vi "basic - Loopback.vi"() -> ()   [LabVIEW 2020]
uses:
  src/AIM664LV.lvlib
  src/_polimorphicInstances/session/Fdx Close Session (Port).vi
  src/_polimorphicInstances/control/Fdx Start (Rx).vi
  src/_polimorphicInstances/session/Fdx Create Session (RX-Monitor).vi
  src/_polimorphicInstances/session/Fdx Create Session (Tx-Generic).vi
  src/_polimorphicInstances/control/Fdx Start (Tx).vi
  src/_polimorphicInstances/control/Fdx Stop (Tx).vi
  src/_polimorphicInstances/control/Fdx Stop (Rx).vi
  src/_controls/session_monitor_config.ctl
  src/_controls/queue_header_generic.ctl
panel:
  out "current time":timestamp
  out "tx timed out":bool
  out "rx timed out":bool
  in  "Data":u8[](array[numeric])=[3, 0, 0, 0, 0, 0, 2, 0, 0, 1, 1, 32, 8, 0, 69, 0, 0, 45, 0, 0, 64, 0, 1, 17, 141, 223, 10, 1, 1, 0, 224, 224, 0, 0, 0, 1, 0, 2, 0, 25, 0, 0, 65, 66, 67, 68, 69, 70, 71, 72, 73, 74, 75, 76, 77, 78, 79, 80, 81, 11] format="%x"
  in  "HeaderInfo":T1={"InterFrameGap"=1000, "PacketGroupWaitTime"=10000, "PayloadBufferMode"=0, "PayloadGenerationMode"=0, "PreambleCount"=0, "Skew"=1, "NetSelect"=4, "FrameStartMode"=1, "PhysErrorInjection"=0, "SequenceNumberInit"=65535, "SequenceNumberOffset"=65535} {"NetSelect" items=["FDX_TX_FRAME_DLY_A"=0, "FDX_TX_FRAME_DLY_B"=1, "FDX_TX_FRAME_BOTH "=3, "FDX_TX_FRAME_ONLY_A"=4, "FDX_TX_FRAME_ONLY_B "=5]; "FrameStartMode" items=["FDX_TX_FRAME_START_IFG", "FDX_TX_FRAME_START_PGWT", "FDX_TX_FRAME_START_TRG"]; "PhysErrorInjection" items=["FDX_TX_FRAME_ERR_OFF"=0, "FDX_TX_FRAME_ERR_CRC"=1, "FDX_TX_FRAME_ERR_ALI"=2, "FDX_TX_FRAME_ERR_PRE"=4, "FDX_TX_FRAME_ERR_PHY"=8]; "SequenceNumberInit" items=["FDX_TX_FRAME_SEQ_INIT_AUTO"=65535]; "SequenceNumberOffset" items=["FDX_TX_FRAME_SEQ_OFFS_AUTO "=65535]; "PayloadGenerationMode" items=["FDX_TX_FRAME_PGM_USER"=0, "FDX_TX_FRAME_PGM_IP_PART"=1, "FDX_TX_FRAME_PGM_IP_FULL"=2, "FDX_TX_FRAME_PGM_IP_PART_TT"=10, "FDX_TX_FRAME_PGM_IP_FULL_TT"=20]; "PayloadBufferMode" items=["FDX_TX_FRAME_PBM_STD", "FDX_TX_FRAME_PBM_MAC", "FDX_TX_FRAME_PBM_UDP"]}
  out "error out":errorcluster
  out "QueueReadOut":T2 {"ReadBuffer" format="%.0x"}
  in  "EntryCount (1)":u32=5
  out "MonStatus":T3 {"MonStatus" items=["FDX_MON_OFF", "FDX_MON_WAIT_FOR_TRIGGER", "FDX_MON_TRIGGERED", "FDX_MON_STOPPED", "FDX_MON_FULL", "FDX_MON_OVERLOAD"]}
  out "GlobalStat Out":T4
  in  "Control":u32(ring)=1 items=["FDX_RX_GS_RES_NO_CNT", "FDX_RX_GS_RES_ALL_CNT", "FDX_RX_GS_RES_ERR_CNT"]
  out "TxStatus":T5
  out "rx link ok":bool
  out "tx link ok":bool
  out "GlobMonSize":u32
  in  "RecordingFileName":path
  in  "MaxFileSize MB (1)":u32=1
  in  "Strobe":u32(ring) items=["FDX_MON_STROBE_DIS", "FDX_MON_STROBE_STOP", "FDX_MON_STROBE_START"]
  in  "CaptureMode":u32(ring) items=["FDX_MON_SINGLE ", "FDX_MON_CONTINUOUS", "FDX_MON_SELECTIVE", "FDX_MON_RECORDING", "FDX_MON_REROS", "FDX_MON_HMU"]
  in  "TriggerPosition":u32
  in  "MonitorConfig":T6 {"DefaultCronoMode" items=["FDX_RX_DEFAULT_ENA_CNT", "FDX_RX_DEFAULT_MON_ENA_ALL", "FDX_RX_DEFAULT_MON_ENA_GOOD"]}
  in  "Rx Port":u32=1
  in  "Rx Board":u32
  out "PortInitOut":T7 {"PortConfig" items=["FDX_SINGLE", "FDX_REDUNDANT"]}
  out "TxQueueInfo":cluster{"QueueBaseAddr":u32, "QueueSizeOut":u32}
  in  "Tx Board":u32
  in  "QueueSizeIn":u32
  in  "Tx Port":u32
  # "ARINC 664 Loopback"
  # "Overview: This examples helps to setup the board (or boards) and validate that it can send and receive parameters.\n\nRequirement: One AIM ARINC-664 board with installed AIM ARINC 664 BSP.\nRestrictions: None.\nInstruction:\n1. Select the Board ID (0 if you have only one board in your system) and the port number. If you want to validate between two ports in one device, you can use tx board and Rx Boardd\n2. Run the VI.\n3. See the result in Current IRIG Time"
  # "HW config"
  # "TX Status"
  # "Monitor Config"
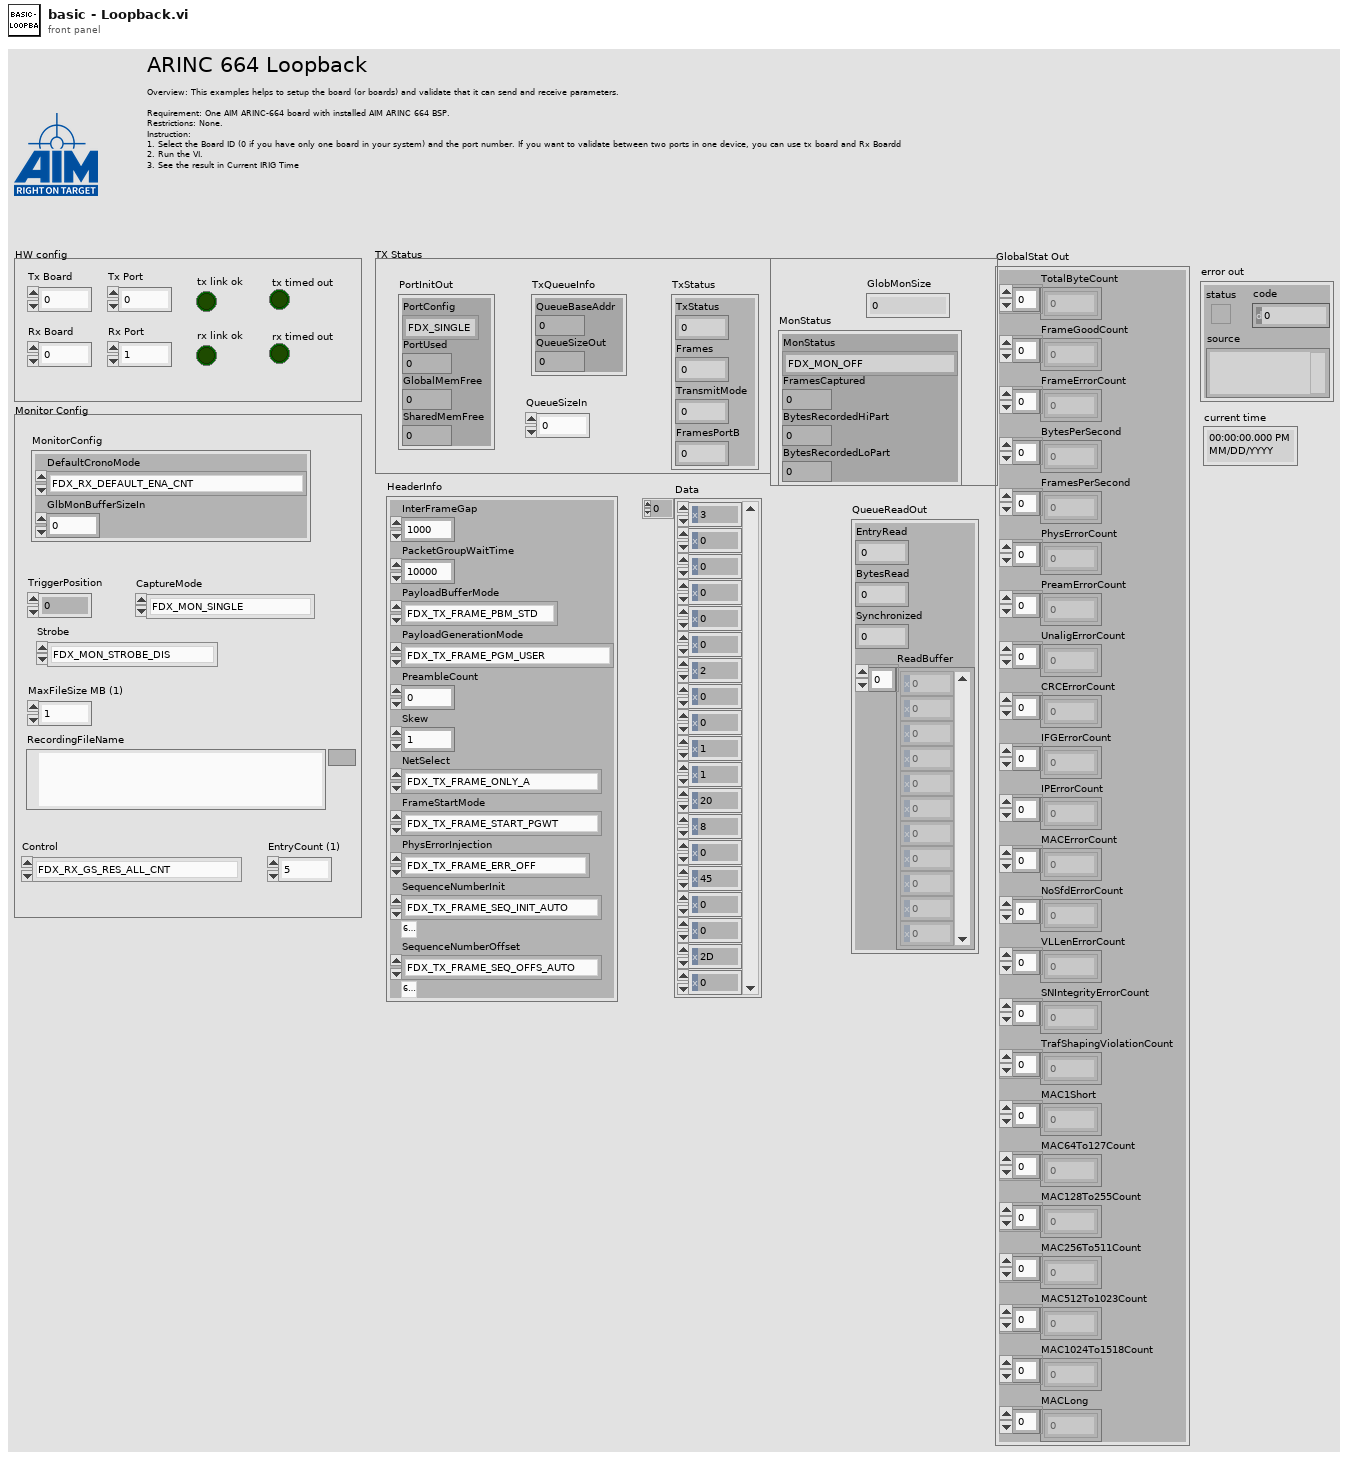
[diagram p1: front panel]
types:
  T1 = typedef "AIM664LV.lvlib/queue_header_generic.ctl" = cluster{"InterFrameGap":u32, "PacketGroupWaitTime":u32, "PayloadBufferMode":u8, "PayloadGenerationMode":u8, "PreambleCount":u8, "Skew":u32, "NetSelect":u8, "FrameStartMode":u8, "PhysErrorInjection":u32, "SequenceNumberInit":u16, "SequenceNumberOffset":u16}
  T2 = cluster{"EntryRead":u32, "BytesRead":u32, "Synchronized":u32, "ReadBuffer":u8[]}
  T3 = cluster{"MonStatus":u32, "FramesCaptured":u32, "BytesRecordedHiPart":u32, "BytesRecordedLoPart":u32}
  T4 = cluster{"TotalByteCount":u32[], "FrameGoodCount":u32[], "FrameErrorCount":u32[], "BytesPerSecond":u32[], "FramesPerSecond":u32[], "PhysErrorCount":u32[], "PreamErrorCount":u32[], "UnaligErrorCount":u32[], "CRCErrorCount":u32[], "IFGErrorCount":u32[], "IPErrorCount":u32[], "MACErrorCount":u32[], "NoSfdErrorCount":u32[], "VLLenErrorCount":u32[], "SNIntegrityErrorCount":u32[], "TrafShapingViolationCount":u32[], "MAC1Short":u32[], "MAC64To127Count":u32[], "MAC128To255Count":u32[], "MAC256To511Count":u32[], "MAC512To1023Count":u32[], "MAC1024To1518Count":u32[], "MACLong":u32[]}
  T5 = cluster{"TxStatus":u32, "Frames":u32, "TransmitMode":u32, "FramesPortB":u32}
  T6 = typedef "AIM664LV.lvlib/session_monitor_config.ctl" = cluster{"DefaultCronoMode":u32, "GlbMonBufferSizeIn":u32}
  T7 = cluster{"PortConfig":u32, "PortUsed":u32, "GlobalMemFree":u32, "SharedMemFree":u32}
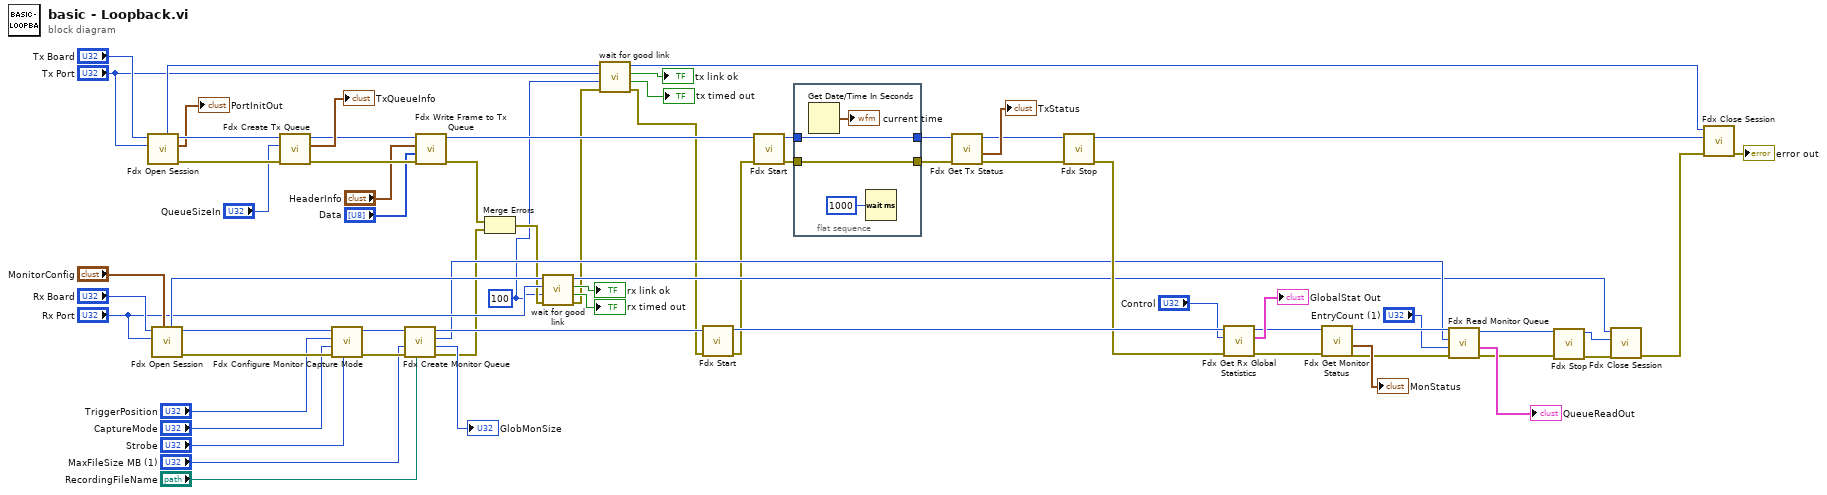
[diagram p0: block diagram]
diagram:
  w2 = u32 100 ("timeout s(10)")
  n1 = call-poly "Fdx Open Session.vi"("port"="Tx Port", "board"="Tx Board") -> ("error out"=w65:errorcluster, "PortInitOut"=→"PortInitOut":T7, "port handle out"=w66:u32, "InstrumentHandle_board out"=w67:u32)  [unwired: 5 in, 1 out]
  n2 = call-poly "Fdx Open Session.vi"("MonitorConfig"="MonitorConfig", "port"="Rx Port", "board"="Rx Board") -> ("error out"=w58:errorcluster, "InstrumentHandle_port out"=w59:u32, "InstrumentHandle_board out"=w49:u32)  [unwired: 3 in, 3 out]
  n3 = call "Fdx Create Tx Queue.vi"("error in (no error)"=w65, "QueueSizeIn"="QueueSizeIn", "InstrumentHandle_port in"=w66) -> ("error out"=w13:errorcluster, "TxQueueInfo"=→"TxQueueInfo":cluster{"QueueBaseAddr":u32, "QueueSizeOut":u32}, "InstrumentHandle_port out"=w15:u32)  [unwired: 6 in]
  n4 = call "Fdx Configure Monitor Capture Mode.vi"("Strobe"="Strobe", "error in (no error)"=w58, "CaptureMode"="CaptureMode", "TriggerPosition"="TriggerPosition", "InstrumentHandle_port in"=w59) -> ("error out"=w53:errorcluster, "InstrumentHandle_port out"=w54:u32)  [unwired: 5 in]
  n5 = call "Fdx Create Monitor Queue.vi"("RecordingFileName"="RecordingFileName", "error in (no error)"=w53, "MaxFileSize MB (1)"="MaxFileSize MB (1)", "InstrumentHandle_port in"=w54) -> ("error out"=w5:errorcluster, "GlobMonSize"=→"GlobMonSize":u32, "QueueIdOut"=w27:u32, "InstrumentHandle_port out"=w43:u32)  [unwired: 4 in]
  n6 = call "Fdx Write Frame to Tx Queue.vi"("error in (no error)"=w13, "Frame in"="Data", "HeaderInfo"="HeaderInfo", "InstrumentHandle_port in"=w15) -> ("error out"=w1:errorcluster, "InstrumentHandle_port out"=w14:u32)  [unwired: 6 in]
  n7 = Merge Errors(w1, w5) -> (w4:errorcluster)
  n8 = call "wait for good link.vi"("error in"=w4, "timeout s(10)"=w2, "port id"="Rx Port", "InstrumentHandle_board in"=w49) -> ("error out"=w6:errorcluster, "timed out"=→"rx timed out":bool, "good link"=→"rx link ok":bool, "InstrumentHandle_board out"=w16:u32)  [unwired: 4 in]
  n9 = call "wait for good link.vi"("error in"=w6, "timeout s(10)"=w2, "port id"="Tx Port", "InstrumentHandle_board in"=w67) -> ("error out"=w3:errorcluster, "timed out"=→"tx timed out":bool, "good link"=→"tx link ok":bool, "InstrumentHandle_board out"=w17:u32)  [unwired: 4 in]
  n10 = call-poly "Fdx Start.vi"("error in (no error)"=w3, "InstrumentHandle_port in"=w43) -> ("error out"=w7:errorcluster, "InstrumentHandle_port out"=w36:u32)  [unwired: 8 in]
  n11 = call-poly "Fdx Start.vi"("error in (no error)"=w7, "InstrumentHandle_port in"=w14) -> ("error out"=w8:errorcluster, "InstrumentHandle_port out"=w42:u32)  [unwired: 8 in]
  n12 = flat-sequence {
    tunnel: w8 -> [w70]
    tunnel: [w70] -> w39
    tunnel: [w69] -> w40
    tunnel: w42 -> [w69]
    frame #0 {
      n13 = Get Date/Time In Seconds() -> (seconds since 1Jan1904=→"current time":timestamp)
      n14 = Wait (ms)(milliseconds to wait=u32 1000) -> ()  [unwired: 1 out]
    }
  }
  n15 = call "Fdx Get Tx Status.vi"("error in (no error)"=w39, "InstrumentHandle_port in"=w40) -> ("error out"=w37:errorcluster, "TxStatus"=→"TxStatus":T5, "InstrumentHandle_port out"=w38:u32)  [unwired: 7 in]
  n16 = call-poly "Fdx Stop.vi"("error in (no error)"=w37, "InstrumentHandle_port in"=w38) -> ("error out"=w34:errorcluster, "InstrumentHandle_port out"=w18:u32)  [unwired: 8 in]
  n17 = call "Fdx Get Rx Global Statistics.vi"("error in (no error)"=w34, "Control"="Control", "InstrumentHandle_port in"=w36) -> ("error out"=w31:errorcluster, "GlobalStat Out"=→"GlobalStat Out":T4, "InstrumentHandle_port out"=w32:u32)  [unwired: 6 in]
  n18 = call "Fdx Get Monitor Status.vi"("error in (no error)"=w31, "InstrumentHandle_port in"=w32) -> ("error out"=w28:errorcluster, "MonStatus"=→"MonStatus":T3, "InstrumentHandle_port out"=w29:u32)  [unwired: 7 in]
  n19 = call "Fdx Read Monitor Queue.vi"("error in (no error)"=w28, "EntryCount (1)"="EntryCount (1)", "QueueId in"=w27, "InstrumentHandle_port in"=w29) -> ("error out"=w23:errorcluster, "QueueReadOut"=→"QueueReadOut":T2, "InstrumentHandle_port out"=w24:u32)  [unwired: 4 in, 1 out]
  n20 = call-poly "Fdx Stop.vi"("error in (no error)"=w23, "InstrumentHandle_port in"=w24) -> ("error out"=w21:errorcluster, "InstrumentHandle_port out"=w22:u32)  [unwired: 8 in]
  n21 = call-poly "Fdx Close Session.vi"("error in (no error)"=w21, "InstrumentHandle_port in"=w22, "InstrumentHandle_board in"=w16) -> ("error out"=w20:errorcluster)  [unwired: 8 in]
  n22 = call-poly "Fdx Close Session.vi"("error in (no error)"=w20, "InstrumentHandle_port in"=w18, "InstrumentHandle_board in"=w17) -> ("error out"=→"error out":errorcluster)  [unwired: 8 in]
